vi "Get Simulated.vi"(8 "error in (no error)":errorcluster, 11 "PS in":refnum<class "PS.lvclass">) -> (0 "error out":errorcluster, 2 "Simulated":bool, 3 "PS out":refnum<class "PS.lvclass">)   [LabVIEW 2020, in "PS.lvclass"]
uses:
  PS.lvclass
  PS.lvclass/PS.ctl
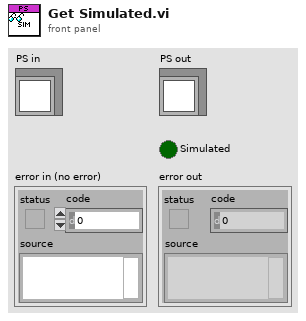
[diagram p1: front panel]
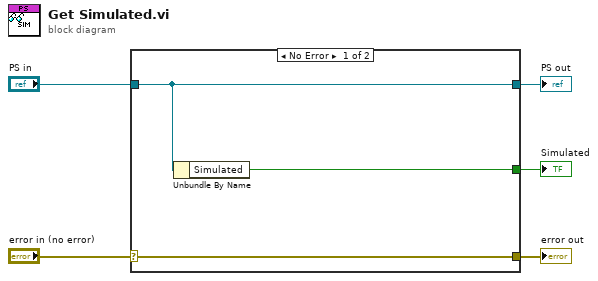
[diagram p0: block diagram]
diagram:
  n1 = case shown="No Error" "error in (no error)" {
    selector: "error in (no error)" -> [w8 w9]
    tunnel: [w8 w9] -> w4
    tunnel: [w7 w10] -> w2
    tunnel: "PS in" -> [w7 w10]
    tunnel: [w6 _] -> w1
    frame No Error {
      n2 = Unbundle By Name(w7) -> ("Simulated"=w6:bool)
    }
    frame Error {
    }
  }
  "error out" <- w4
  "PS out" <- w2
  "Simulated" <- w1
